vi "Get Config.vi"(9 "rf channel selector":T2, 11 "rx.coerced configurations":T1) -> (2 "file preamble":string)   [LabVIEW 2018]
uses:
  typedefs/rf.channel selector.ctl
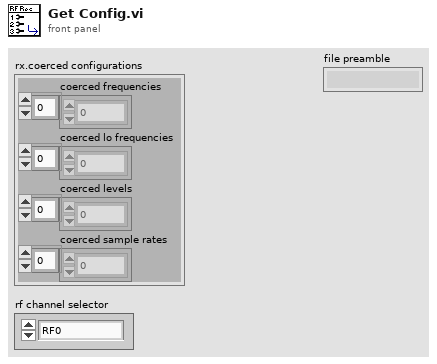
[diagram p1: front panel]
types:
  T1 = cluster{"coerced frequencies":dbl[], "coerced lo frequencies":dbl[], "coerced levels":dbl[], "coerced sample rates":dbl[]}
  T2 = typedef "rf.channel selector.ctl" = enum16{"RF0", "RF1"}
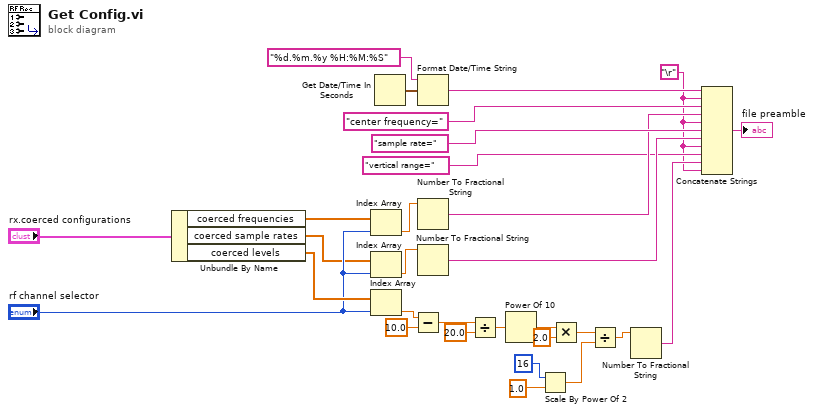
[diagram p0: block diagram]
diagram:
  w7 = "\r"
  n1 = Unbundle By Name("rx.coerced configurations") -> ("coerced frequencies"=w20:dbl[], "coerced sample rates"=w21:dbl[], "coerced levels"=w23:dbl[])
  n2 = Index Array(array=w20, index="rf channel selector") -> (element=w25:dbl)
  n3 = Index Array(array=w21, index="rf channel selector") -> (element=w28:dbl)
  n4 = Index Array(array=w23, index="rf channel selector") -> (element=w27:dbl)
  n5 = Get Date/Time In Seconds() -> (seconds since 1Jan1904=w10:timestamp)
  n6 = Subtract(x=w27, y=10.0) -> (x-y=w17:dbl)
  n7 = Format Date/Time String(time format string (%c)="%d.%m.%y %H:%M:%S", seconds (now)=w10) -> (date/time string=w12:string)  [unwired: 1 in]
  n8 = Number To Fractional String(number=w25) -> (F-format string=w26:string)  [unwired: 3 in]
  n9 = Number To Fractional String(number=w28) -> (F-format string=w30:string)  [unwired: 3 in]
  n10 = Divide(x=w17, y=20.0) -> (x/y=w18:dbl)
  n11 = Power Of 10(x=w18) -> (10^x=w19:dbl)
  n12 = Scale By Power Of 2(n=i16 16 ("ADC Resolution (bits)"), x=1.0) -> (x*2^n=w1:dbl)
  n13 = Multiply(x=w19, y=2.0) -> (x*y=w2:dbl)
  n14 = Divide(x=w2, y=w1) -> (x/y=w3:dbl)
  n15 = Number To Fractional String(number=w3) -> (F-format string=w8:string)  [unwired: 3 in]
  n16 = Concatenate Strings(w12, w7, "center frequency=" ("string"), w26, w7, "sample rate=" ("string"), w30, w7, "vertical range=" ("string"), w8, w7) -> (→"file preamble":string)
